vi "Parse XML to DS.vi"(0 "Refnum in":refnum<k20>, 1 "LV Proj File Path":path, 5 "Node Name":string, 7 "Item Indent":i32) -> (4 "DS":T1(array[cluster]), 6 "Node Names":string[](array[string]))   [LabVIEW 2016]
uses:
  <vilib>/xml/Load XML File.vi
  <vilib>/xml/Close Reference(Node).vi
  <vilib>/xml/Close Reference(NNMap).vi
  <resource>/objmgr/DOMUserDefRef.rc
  <vilib>/xml/NI_XML.lvlib
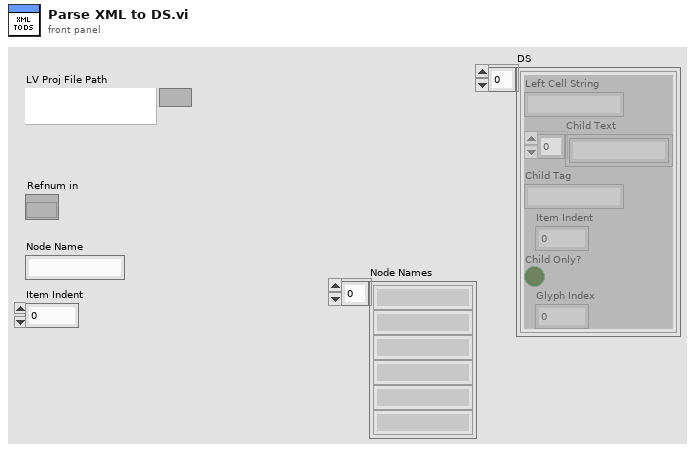
[diagram p1: front panel]
types:
  T1 = cluster{"Left Cell String":string, "Child Text":string[], "Child Tag":string, "Item Indent":i32, "Child Only?":bool, "Glyph Index":i32}[]
  T2 = cluster{"Left Cell String":string, "Child Text":string[], "Child Tag":string, "Item Indent":i32, "Child Only?":bool, "Glyph Index":i32}
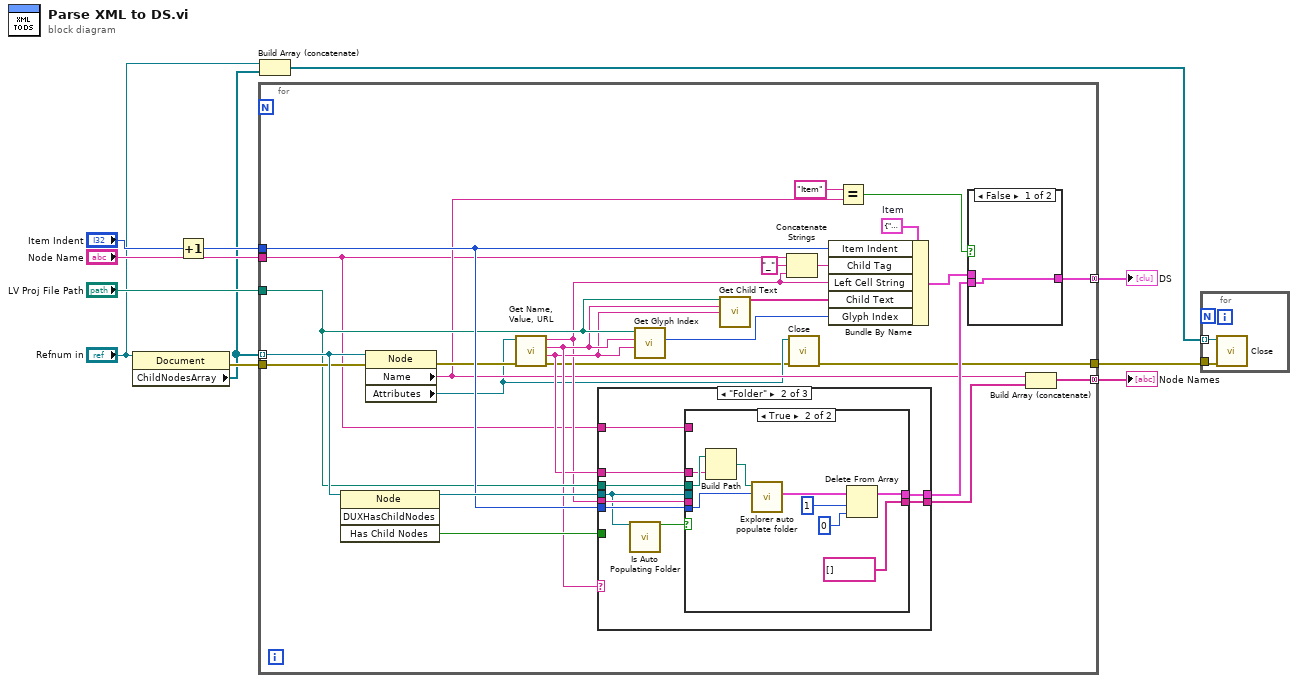
[diagram p0: block diagram]
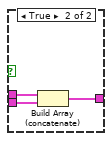
[diagram p2: hidden frame]
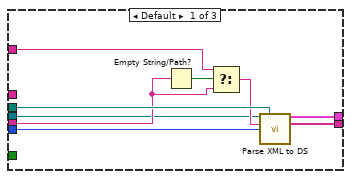
[diagram p3: hidden frame]
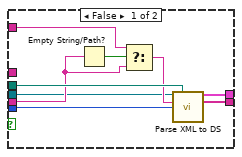
[diagram p4: hidden frame]
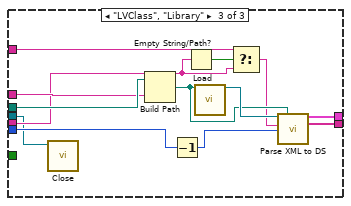
[diagram p5: hidden frame]
diagram:
  n1 = property class="Document"(reference="Refnum in") -> (error out=w6:errorcluster, "ChildNodesArray"=w3:refnum<k20>[])  [unwired: 1 in, 1 out]
  n2 = Increment(x="Item Indent") -> (x+1=w8:i32)
  n3 = for {
    tunnel: w3 -> [w38] mode=indexing
    tunnel: [w35] -> w11 mode=concatenating
    tunnel: "Node Name" -> [w17]
    tunnel: w8 -> [w32]
    tunnel: [w31] -> w7 mode=concatenating
    tunnel: w6 -> [w26]
    tunnel: [w13] -> w4
    tunnel: "LV Proj File Path" -> [w23]
    w34 = T2 {"Left Cell String"="", "Child Text"=[], "Child Tag"="", "Item Indent"=0, "Child Only?"=FALSE, "Glyph Index"=0}  # Item
    n4 = invoke class="Node" method="DUXHasChildNodes"(reference=w38) -> (reference out=w36:refnum<k20>, "Has Child Nodes"=w37:bool)  [unwired: 3 in, 2 out]
    n5 = property class="Node"(reference=w38, error in=w26) -> (error out=w25:errorcluster, "Name"=w18:string, "Attributes"=w15:refnum<k20>)  [unwired: 1 out]
    n6 = call "Get Name, Value, URL.vi"("error in (no error)"=w25, "Refnum in"=w15) -> ("error out"=w14:errorcluster, "URL"=w21:string, "Type"=w22:string, "Name"=w20:string)  [unwired: 6 in]
    n7 = case shown="\"Folder\"" w22 {
      tunnel: w36 -> [w43 w54 w84]
      tunnel: w20 -> [w45 w55 w86]
      tunnel: w32 -> [w51 w60 w87]
      tunnel: [w50 w59 w91] -> w30
      tunnel: [w49 w58 w90] -> w29
      tunnel: w23 -> [w48 w57 w89]
      tunnel: w21 -> [_ w52 w88]
      tunnel: w17 -> [w46 w56 w85]
      tunnel: w37 -> [_ _ _]
      frame Default {
        n8 = Empty String/Path?(string/path=w45) -> (empty?=w47:bool)
        n9 = Select(t=w46, s=w47, f=w45) -> (s? t:f=w44:string)
        n10 = call "Parse XML to DS.vi"("Refnum in"=w43, "LV Proj File Path"=w48, "Node Name"=w44, "Item Indent"=w51) -> ("DS"=w49:T1, "Node Names"=w50:string[])  [unwired: 10 in]
      }
      frame "Folder" {
        n11 = call "Is Auto Populating Folder.vi"("Refnum in"=w54) -> ("Auto Populating Folder?"=w53:bool)  [unwired: 14 in]
        n12 = case shown="True" w53 {
          tunnel: w60 -> [w69 w74]
          tunnel: [w68 string[] [] ("Array 2")] -> w59
          tunnel: [w67 w72] -> w58
          tunnel: w57 -> [w66 w77]
          tunnel: w56 -> [w64 _]
          tunnel: w55 -> [w63 _]
          tunnel: w54 -> [w61 _]
          tunnel: w52 -> [_ w76]
          frame False {
            n13 = Empty String/Path?(string/path=w63) -> (empty?=w65:bool)
            n14 = Select(t=w64, s=w65, f=w63) -> (s? t:f=w62:string)
            n15 = call "Parse XML to DS.vi"("Refnum in"=w61, "LV Proj File Path"=w66, "Node Name"=w62, "Item Indent"=w69) -> ("DS"=w67:T1, "Node Names"=w68:string[])  [unwired: 10 in]
          }
          frame True {
            n16 = Build Path(base path=w77, name or relative path=w76) -> (appended path=w75:path)
            n17 = call "Explorer auto populate folder.vi"("Item Indent"=w74, "Folder Path"=w75) -> ("Items"=w73:T1)  [unwired: 7 in, 2 out]
            n18 = Delete From Array(array=w73, length=1, index=0) -> (array with subset deleted=w72:T1)  [unwired: 1 out]
          }
        }
      }
      frame "LVClass", "Library" {
        n19 = call-poly <vilib>:"Close.vi"("node"=w84) -> ()  [unwired: 8 in, 1 out]
        n20 = Build Path(base path=w89, name or relative path=w88) -> (appended path=w82:path)
        n21 = Decrement(x=w87) -> (x-1=w81:i32)
        n22 = Empty String/Path?(string/path=w86) -> (empty?=w80:bool)
        n23 = call-poly <vilib>:"Load.vi"("path to XML document"=w82) -> ("DOM document out"=w83:refnum<k20>)  [unwired: 12 in, 2 out]
        n24 = Select(t=w85, s=w80, f=w86) -> (s? t:f=w79:string)
        n25 = call "Parse XML to DS.vi"("Refnum in"=w83, "LV Proj File Path"=w82, "Node Name"=w79, "Item Indent"=w81) -> ("DS"=w90:T1, "Node Names"=w91:string[])  [unwired: 10 in]
      }
    }
    n26 = call "Get Glyph Index.vi"("URL"=w21, "Type"=w22, "LV Proj File Path"=w23) -> ("Glyph Index"=w12:i32)  [unwired: 8 in]
    n27 = call "Get Child Text.vi"("Item File Path"=w23, "Node Type"=w22, "Node URL"=w21) -> ("Child Text"=w24:string[])  [unwired: 12 in]
    n28 = Concatenate Strings(w17, "_" ("string"), w20) -> (w33:string)
    n29 = call-poly <vilib>:"Close.vi"("error in (no error)"=w14, "named node map"=w15) -> ("error out"=w13:errorcluster)  [unwired: 7 in]
    n30 = Bundle By Name(cluster=w34, "Item Indent"=w32, "Child Tag"=w33, "Left Cell String"=w20, "Child Text"=w24, "Glyph Index"=w12) -> (w16:T2)
    n31 = Equal?(x="Item", y=w18) -> (x = y?=w27:bool)
    n32 = case shown="False" w27 {
      tunnel: w16 -> [_ w42]
      tunnel: [w39 w41] -> w31
      tunnel: w29 -> [w39 w40]
      frame False {
      }
      frame True {
        n33 = Build Array (concatenate)(w42, w40) -> (w41:T1)
      }
    }
    n34 = Build Array (concatenate)(w18, w30) -> (w35:string[])
  }
  "Node Names" <- w11
  "DS" <- w7
  n35 = Build Array (concatenate)("Refnum in", w3) -> (w1:refnum<k20>[])
  n36 = for {
    tunnel: w4 -> [w93]
    tunnel: w1 -> [w92] mode=indexing
    n37 = call-poly <vilib>:"Close.vi"("error in (no error)"=w93, "node"=w92) -> ()  [unwired: 7 in, 1 out]
  }
